vi "arm-execute-sim.vi"   [LabVIEW 2020]
uses:
  RobotCode/Arm/ArmGlobal.vi
  arm-sim-globals.vi
  RobotCode/Human/HumanGlobal.vi
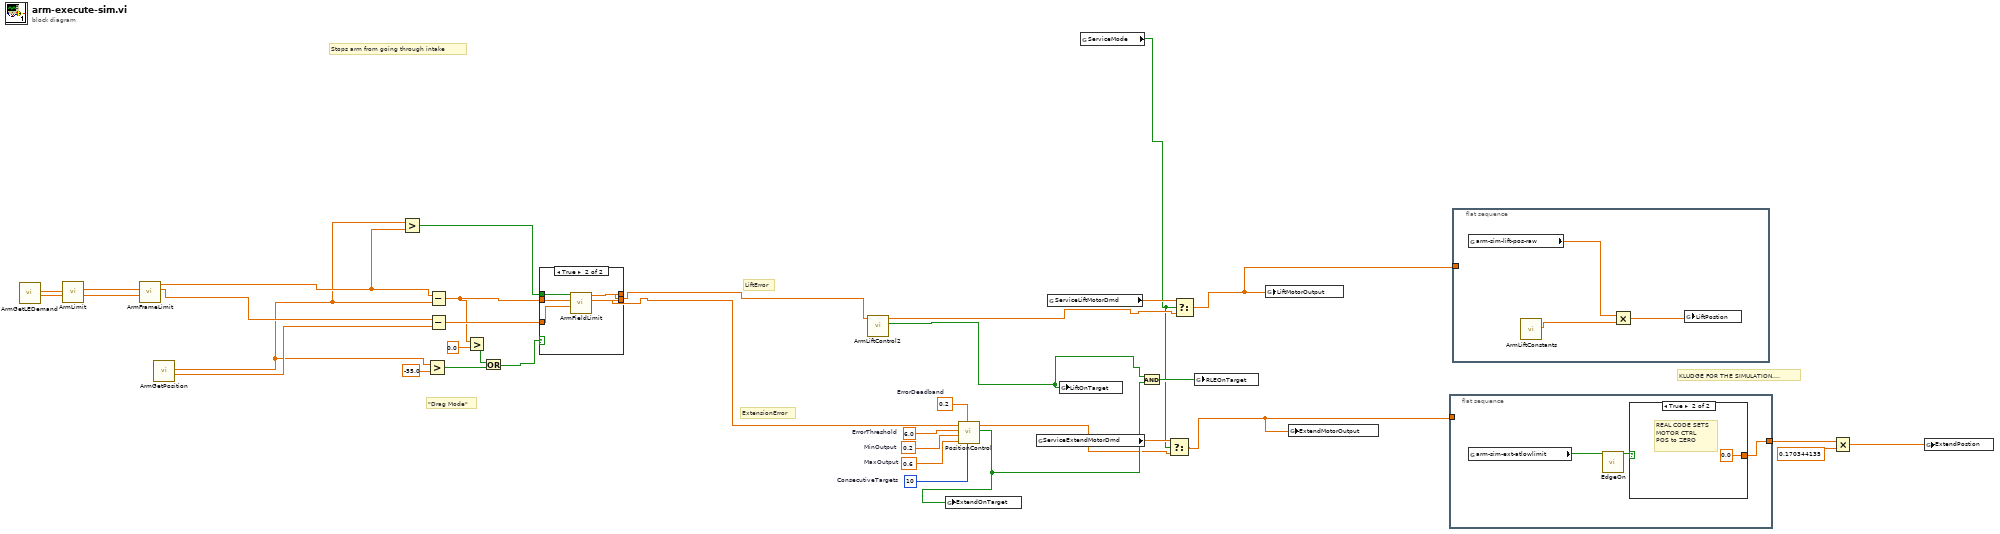
[diagram p0: block diagram]
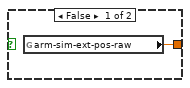
[diagram p3: hidden frame]
diagram:
  w29 = 10  # ConsecutiveTargets
  w30 = 0.6  # MaxOutput
  w31 = 0.2  # MinOutput
  w32 = 6.0  # ErrorThreshold
  w33 = 0.2  # ErrorDeadband
  # "\"Drag Mode\""
  # "Stops arm from going through intake"
  # "ExtensionError"
  # "LiftError"
  # "KLUDGE FOR THE SIMULATION...."
  n1 = call "ArmGetLEDemand.vi"() -> ("ExtendPositonDemand(in)"=w25:dbl, "LiftPositionDemand(d)"=w26:dbl)  [unwired: 10 in]
  n2 = call "ArmLimit.vi"("Extend"=w25, "Lift"=w26) -> ("Extend"=w12:dbl, "Lift"=w13:dbl)  [unwired: 8 in]
  n3 = call "ArmFrameLimit.vi"("Extend Setpoint"=w12, "Lift Setpoint"=w13) -> ("Extend Position"=w10:dbl, "Lift Setpoint"=w11:dbl)  [unwired: 8 in]
  n4 = call "ArmGetPosition.vi"() -> ("ExtendPostion"=w17:dbl, "LiftPostion"=w8:dbl)  [unwired: 10 in]
  n5 = Greater?(x=w8, y=w11) -> (0:w16:bool)
  n6 = Greater?(x=w8, y=-55.0) -> (0:w6:bool)
  n7 = Subtract(x=w11, y=w8) -> (x-y=w3:dbl)
  n8 = Subtract(x=w10, y=w17) -> (x-y=w18:dbl)
  n9 = Greater?(x=w3, y=0.0) -> (0:w4:bool)
  n10 = Or(x=w4, y=w6) -> (x .or. y?=w7:bool)
  n11 = case shown="True" w7 {
    tunnel: w18 -> [w37 w43]
    tunnel: w3 -> [w38 w42]
    tunnel: w16 -> [_ w41]
    tunnel: [w38 w40] -> w15
    tunnel: [w37 w39] -> w14
    frame False {
    }
    frame True {
      n12 = call "ArmFieldLimit.vi"("Extend Error"=w43, "Lift Error"=w42, "Going Down?"=w41) -> ("Extend Error"=w39:dbl, "Lift Error"=w40:dbl)  [unwired: 7 in]
    }
  }
  n13 = call "ArmLiftControl2.vi"("erronIn(d)"=w15) -> ("OnTarget"=w19:bool, "motorOutput"=w23:dbl)  [unwired: 9 in]
  n14 = call "PositionControl.vi"("ConsecutiveTargets"=w29, "ErrorDeadband"=w33, "MaxOutput"=w30, "MinOutput"=w31, "ErrorThreshold"=w32, "Error"=w14) -> ("OnTarget"=w28:bool, "OutputValue"=w21:dbl)  [unwired: 3 in, 1 out]
  n15 = global write "ArmGlobal.vi" "ExtendOnTarget"(w28) -> ()
  n16 = global read "HumanGlobal.vi" "ServiceExtendMotorDmd"() -> (w22:dbl)
  n17 = global read "HumanGlobal.vi" "ServiceLiftMotorDmd"() -> (w24:dbl)
  n18 = global write "ArmGlobal.vi" "LiftOnTarget"(w19) -> ()
  n19 = global read "HumanGlobal.vi" "ServiceMode"() -> (w20:bool)
  n20 = And(x=w19, y=w28) -> (x .and. y?=w27:bool)
  n21 = Select(t=w22, s=w20, f=w21) -> (s? t:f=w1:dbl)
  n22 = Select(t=w24, s=w20, f=w23) -> (s? t:f=w2:dbl)
  n23 = global write "ArmGlobal.vi" "RLEOnTarget"(w27) -> ()
  n24 = global write "ArmGlobal.vi" "LiftMotorOutput"(w2) -> ()
  n25 = global write "ArmGlobal.vi" "ExtendMotorOutput"(w1) -> ()
  n26 = flat-sequence {
    tunnel: [w45] -> w34
    tunnel: w1 -> [_]
    frame #0 {
      n27 = global read "arm-sim-globals.vi" "arm-sim-ext-atlowlimit"() -> (w44:bool)
      n28 = call "EdgeOn.vi"("Current State"=w44) -> ("Edge On Found"=w46:bool)  [unwired: 10 in]
      n29 = case shown="True" w46 {
        tunnel: [w47 0.0 ("arm-sim-ext-pos-raw")] -> w45
        frame False {
          n30 = global read "arm-sim-globals.vi" "arm-sim-ext-pos-raw"() -> (w47:dbl)
        }
        frame True {
          # "REAL CODE SETS\nMOTOR CTRL\nPOS to ZERO"
        }
      }
    }
  }
  n31 = flat-sequence {
    tunnel: w2 -> [_]
    frame #0 {
      n32 = global read "arm-sim-globals.vi" "arm-sim-lift-pos-raw"() -> (w49:dbl)
      n33 = call "ArmLiftConstants.vi"() -> ("LiftConversionFactor"=w50:dbl)  [unwired: 8 in, 3 out]
      n34 = Multiply(x=w49, y=w50) -> (x*y=w51:dbl)
      n35 = global write "ArmGlobal.vi" "LiftPostion"(w51) -> ()
    }
  }
  n36 = Multiply(x=w34, y=0.170344135) -> (x*y=w35:dbl)
  n37 = global write "ArmGlobal.vi" "ExtendPostion"(w35) -> ()
